vi "ejercicio 7.vi"() -> ()   [LabVIEW 2015]
panel:
  in  "Detener":bool
  in  "Velocidad":dbl(slide) scale=0.0..200.0
  out "Waveform Chart":dynamicdata(graph)
  in  "Calve":string
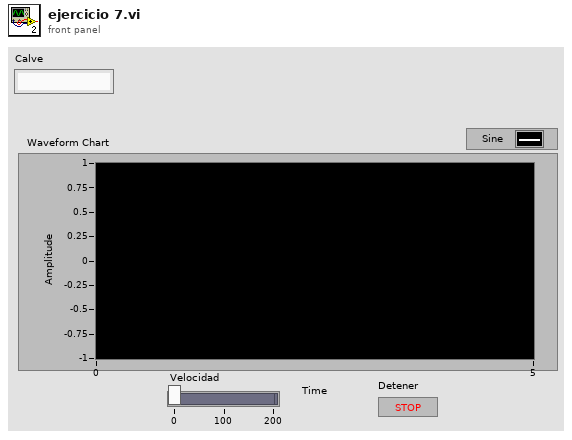
[diagram p1: front panel]
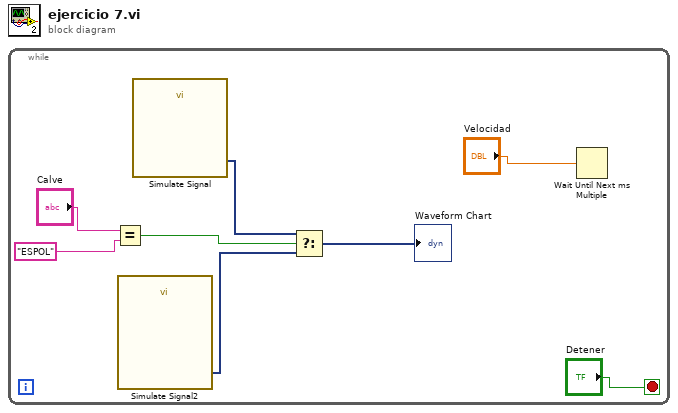
[diagram p0: block diagram]
diagram:
  n1 = while {
    stop <- "Detener" stop-if-true
    n2 = Equal?(x="Calve", y="ESPOL") -> (x = y?=w4:bool)
    n3 = call "Simulate Signal2"() -> ("Triangle"=w7:dynamicdata)  [unwired: 14 in, 1 out]
    n4 = call "Simulate Signal"() -> ("Sine"=w6:dynamicdata)  [unwired: 14 in, 1 out]
    n5 = Select(t=w6, s=w4, f=w7) -> (s? t:f=→"Waveform Chart":dynamicdata)
    n6 = Wait Until Next ms Multiple(millisecond multiple="Velocidad") -> ()  [unwired: 1 out]
  }
